vi "Is One Frontmost__ogtk.vi"(8 "error in":errorcluster caption="error in (no error)", 10 "VI names":string[](array[string])) -> (0 "error out":errorcluster, 1 "VI Refnum":refnum<vi>, 2 "yes":bool, 3 "VI name":string)   [LabVIEW 2016]
doc: "Tests whether the front panel of any of the specified VIs is currently the frontmost window. If so, a reference to that VI is returned.\n\nGenerates no errors.\n\nCopyright © 2003 by Paul F. Sullivan. All rights reserved. You are only permitted the usage indicated in your license agreement."
panel:
  # "Is One Frontmost.vi\n\nTests whether the front panel of any of the specified VIs is currently the frontmost window. If so, a reference to that VI is returned.\n\nPlease visit http://www.OpenG.org to learn about the\nOpen Source LabVIEW software movement.\n\nNOTICE -- YOU MUST LEAVE THIS NOTICE IN PLACE.  PER THE TERMS OF THE LICENSE BELOW, YOU MAY SUBLICENSE THIS SOFTWARE \nIN ANY WAY THAT DOES NOT CONFLICT WITH THIS LICENSE.\n\n### BSD License (http://www.opensource.org/licenses/bsd-license.php) Begin ###\n \nCopyright (c) 2003, Paul F. Sullivan <Paul@SULLutions.com>\nCopyright (c) 2004, Jim Kring <jim@jimkring.com>\n\nAll rights reserved.\n\nRedistribution and use in source and binary forms, with or without modification, are permitted provided that the following conditions are met:\n\n    * Redistributions of source code must retain the above copyright notice, this list of conditions and the following disclaimer.\n    * Redistributions in binary form must reproduce the above copyright notice, this list of conditions and the following disclaimer in the \n       documentation and/or other materials provided with the distribution.\n    * Neither the name of SciWare, James Kring, Inc., nor the names of its contributors may be used to endorse or promote products derived \n       from this software without specific prior written permission.\n\nTHIS SOFTWARE IS PROVIDED BY THE COPYRIGHT HOLDERS AND CONTRIBUTORS \"AS IS\" AND ANY EXPRESS OR IMPLIED WARRANTIES, \nINCLUDING, BUT NOT LIMITED TO, THE IMPLIED WARRANTIES OF MERCHANTABILITY AND FITNESS FOR A PARTICULAR PURPOSE ARE \nDISCLAIMED. IN NO EVENT SHALL THE COPYRIGHT OWNER OR CONTRIBUTORS BE LIABLE FOR ANY DIRECT, INDIRECT, INCIDENTAL,\n SPECIAL, EXEMPLARY, OR CONSEQUENTIAL DAMAGES (INCLUDING, BUT NOT LIMITED TO, PROCUREMENT OF SUBSTITUTE GOODS OR \nSERVICES; LOSS OF USE, DATA, OR PROFITS; OR BUSINESS INTERRUPTION) HOWEVER CAUSED AND ON ANY THEORY OF LIABILITY, \nWHETHER IN CONTRACT, STRICT LIABILITY, OR TORT (INCLUDING NEGLIGENCE OR OTHERWISE) ARISING IN ANY WAY OUT OF THE USE \nOF THIS SOFTWARE, EVEN IF ADVISED OF THE POSSIBILITY OF SUCH DAMAGE.\n\n### BSD License End ###"
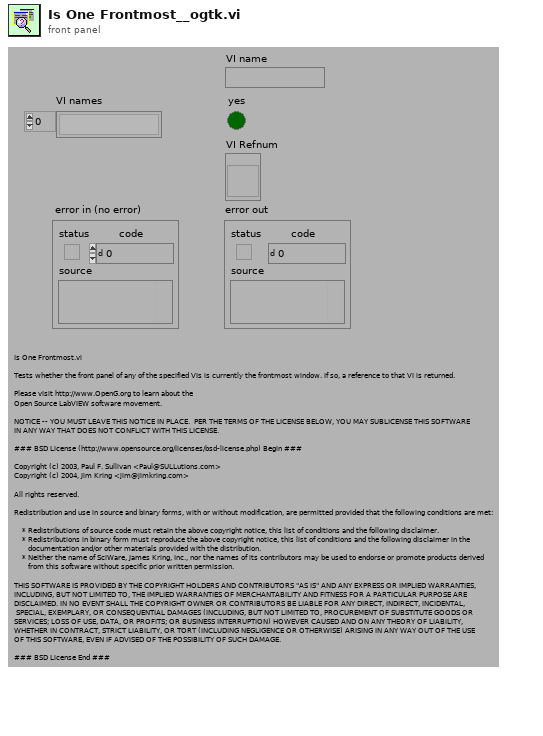
[diagram p1: front panel]
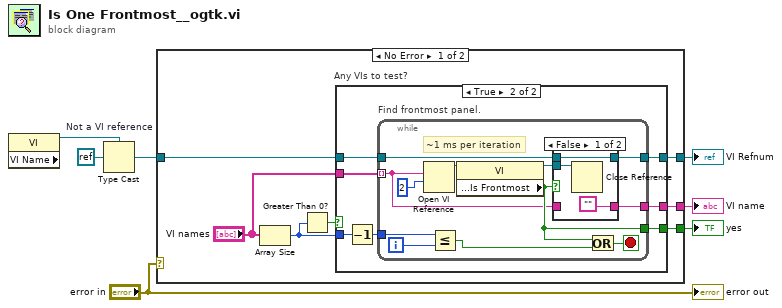
[diagram p0: block diagram]
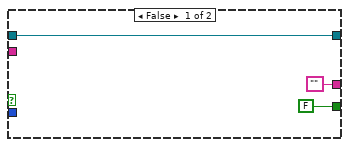
[diagram p2: hidden frame]
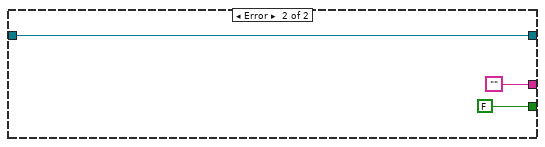
[diagram p4: hidden frame]
diagram:
  n1 = property class="VI" props=["VI Name"]() -> (reference out=w3:refnum<vi>)  [unwired: 2 in, 2 out]
  n2 = Type Cast "Not a VI reference"(type=w3, x=refnum<k0> refnum) -> (*(type *) &x=w2:refnum<vi>)
  n3 = case shown="No Error" "error in" {
    tunnel: [w14 w44] -> w6
    tunnel: [w13 FALSE] -> w5
    tunnel: w2 -> [w11 w44]
    tunnel: [w8 ""] -> w1
    frame No Error {
      n4 = Array Size(array="VI names") -> (size(s)=w9:i32)
      n5 = Greater Than 0?(x=w9) -> (x > 0?=w10:bool)
      n6 = case "Any VIs to test?" shown="True" w10 {
        tunnel: [w17 w24] -> w14
        tunnel: [FALSE ("Front Panel.IsFrontmost") w23] -> w13
        tunnel: w9 -> [_ w21]
        tunnel: "VI names" -> [_ w20]
        tunnel: w11 -> [w17 w19]
        tunnel: ["" w18] -> w8
        frame False {
        }
        frame True {
          n7 = Decrement(x=w21) -> (x-1=w22:i32)
          n8 = while "Find frontmost panel." {
            tunnel: [w26] -> w18
            tunnel: w19 -> [w28]
            tunnel: [w29] -> w23
            tunnel: [w32] -> w24
            tunnel: w22 -> [w34]
            tunnel: w20 -> [w27] mode=indexing
            i -> [w35]
            stop <- w31 stop-if-true
            # "~1 ms per iteration"
            n9 = Open VI Reference(vi path=w27, options=2) -> (vi reference=w36:refnum<vi>)  [unwired: 4 in, 1 out]
            n10 = Less Or Equal?(x=w34, y=w35) -> (x <= y?=w30:bool)
            n11 = property class="VI"(reference=w36) -> (reference out=w33:refnum<vi>, "Front Panel Window:Is Frontmost"=w29:bool)  [unwired: 1 in, 1 out]
            n12 = case shown="False" w29 {
              tunnel: w33 -> [w39 w41]
              tunnel: [w38 w41] -> w32
              tunnel: w28 -> [w38 _]
              tunnel: w27 -> [_ w40]
              tunnel: ["" w40] -> w26
              frame False {
                n13 = Close Reference(reference=w39) -> ()  [unwired: 1 in, 1 out]
              }
              frame True {
              }
            }
            n14 = Or(x=w29, y=w30) -> (x .or. y?=w31:bool)
          }
        }
      }
    }
    frame Error {
    }
  }
  "yes" <- w5
  "VI Refnum" <- w6
  "VI name" <- w1
  "error out" <- "error in"
